vi "Main VERSION 1.1.vi"() -> ()   [LabVIEW 2017]
uses:
  <vilib>/Math Plots/3D Math Plots/3D Surface/3D Surface XCtrl/3D Surface.xctl
  <vilib>/Math Plots/3D Math Plots/3D Surface/3D Surface Datatype/3D Surface Datatype.lvclass
  CSV Reader Inputs.ctl
  Frequency_Type.ctl
  Measurement_Type.ctl
  Digital Channel Selector.ctl
  State.ctl
  Data.ctl
  <vilib>/Platform/TimedLoop/XDataNode/timing_clust.ctl
  <vilib>/Platform/TimedLoop/XDataNode/nitl_modes.ctl
  <vilib>/Platform/TimedLoop/XDataNode/wakeup.ctl
  <vilib>/addons/Control Design/_Model Construction/Data Typedefs.llb/CD DtoC Conversion Method.ctl
  <vilib>/imath/engines/lvmath2/RunTimeEngine/Managers/WorkSpace/UID Generator.vi
  <vilib>/imath/engines/lvmath2/RunTimeEngine/BuiltInFunctions/zpk_to_tf/NIMS_zpk_to_tf.vi
  <vilib>/imath/engines/lvmath2/RunTimeEngine/RunTimeType/NIMS_RunTimeType_From StrictType (excl LVString).vi
  <instcachedir>/0/NIMS_RunTimeType_From StrictType (excl LVString)_DC56D72BB6B948F98D63F1A957D87C42.lvgen/NIMS_RunTimeType_From StrictType (excl LVString)_DC56D72BB6B948F98D63F1A957D87C42_000.vi
  <vilib>/imath/engines/lvmath2/RunTimeEngine/ErrorHandling/NIMS_Error From Error Code.vi
  <vilib>/imath/engines/lvmath2/RunTimeEngine/LocalVariableDefStatement/MC_LocalVariableDefStatement_Display.vi
  <vilib>/imath/engines/lvmath2/RunTimeEngine/Managers/SymbolTable/Clear UID.vi
  <vilib>/imath/engines/lvmath2/RunTimeEngine/NodeEndStatement/NIMS_NodeEndStatement_Output.vi
  <instcachedir>/0/NIMS_NodeEndStatement_Output_53EC0D466D134D7ABD903AC30B43404B.lvgen/NIMS_NodeEndStatement_Output_53EC0D466D134D7ABD903AC30B43404B_005.vi
  <vilib>/imath/engines/lvmath2/RunTimeEngine/ErrorHandling/NIMS_Finalize Error.vi
  <vilib>/addons/Control Design/_Model Construction/Model Creation.llb/Model Creation SubVI/cd_Create Transfer Function Model.vi
  <vilib>/addons/Control Design/_Model Construction/Model Information.llb/Model Information SubVIs/cd_Set Names To TF Model.vi
  <vilib>/addons/Control Design/_Utility/Model Viewer.llb/Model Viewer SubVI/cd_Draw Transfer Function Equation (TF).vi
  <vilib>/addons/Control Design/_Time Response Analysis/Time Response.llb/Time Response subVI/cd_Linear Simulation (Transfer Function).vi
  <vilib>/addons/Control Design/_Dynamic Analysis/Dynamic Analysis.llb/Dynamic Analysis subVI/cd_Damping Ratio and Natural Frequency (Transfer Function).vi
  <vilib>/addons/Wavelet Analysis/application.llb/WA Detrend (Waveform).vi
  Program Files (x86)/National Instruments/LabVIEW 2017/vi.lib/addons/System Identification/Data Preprocess.llb/SI Lowpass Filter (SISO Waveform).vi
  <vilib>/addons/Time Series Analysis/Modeling and Prediction.llb/TSA ARMA Modeling (Waveform).vi
  <vilib>/addons/Control Design/_Model Conversions/Continuous and Discrete.llb/Continuous and Discrete SubVI/cd_Convert Discrete to Continuous (TF).vi
  <vilib>/addons/Control Design/_Model Conversions/Model Type.llb/Model Conversion SubVI/cd_Convert Transfer Function to State-Space Model.vi
  <vilib>/addons/Control Design/_Dynamic Analysis/Dynamic Analysis.llb/Dynamic Analysis subVI/cd_Damping Ratio and Natural Frequency (State-Space).vi
  <vilib>/imath/engines/lvmath2/RunTimeEngine/BuiltInFunctions/sort/NIMS_[2o]_sort(RRowV,I32,Str).vi
  <instcachedir>/0/NIMS_[2o]_sort(RRowV,I32,Str)_E84E23B068DF4763991B1E74560868DE.lvgen/NIMS_[2o]_sort(RRowV,I32,Str)_E84E23B068DF4763991B1E74560868DE_000.vi
  <vilib>/imathl/engines/lvmath/Functions/Error Handling/Create Error.vi
  <vilib>/imath/engines/lvmath2/RunTimeEngine/IndexRead/NIMS V(V).vi
  <instcachedir>/0/NIMS V(V)_298D9CB7BFEB42B8BC8D9C3C28AE8C70.lvgen/NIMS V(V)_298D9CB7BFEB42B8BC8D9C3C28AE8C70_000.vi
  <instcachedir>/0/NIMS V(V)_298D9CB7BFEB42B8BC8D9C3C28AE8C70.lvgen/NIMS V(V)_298D9CB7BFEB42B8BC8D9C3C28AE8C70_001.vi
  <vilib>/imath/engines/lvmath2/RunTimeEngine/BitwiseOperatorToken/NIMS_Bitwise_Operator_And.vi
  <instcachedir>/0/NIMS_Bitwise_Operator_And_BF79565AECDF4B89921EA9614C6BB008.lvgen/NIMS_Bitwise_Operator_And_BF79565AECDF4B89921EA9614C6BB008_001.vi
  <vilib>/imath/engines/lvmath2/RunTimeEngine/BuiltInFunctions/imag/NIMS_imag(Complex).vi
  <instcachedir>/0/NIMS_imag(Complex)_3180D40D00C843A49C2B33397F857BF3.lvgen/NIMS_imag(Complex)_3180D40D00C843A49C2B33397F857BF3_002.vi
  <vilib>/imath/engines/lvmath2/RunTimeEngine/BuiltInFunctions/findnz/NIMS_[1o]_findnz(GRowV).vi
  <instcachedir>/0/NIMS_[1o]_findnz(GRowV)_4566141FE5BA40B7B10E18ED0AB78B2D.lvgen/NIMS_[1o]_findnz(GRowV)_4566141FE5BA40B7B10E18ED0AB78B2D_000.vi
  <vilib>/imath/engines/lvmath2/RunTimeEngine/ErrorHandling/NIMS_Create Error From Enums.vi
  <instcachedir>/0/NIMS_NodeEndStatement_Output_53EC0D466D134D7ABD903AC30B43404B.lvgen/NIMS_NodeEndStatement_Output_53EC0D466D134D7ABD903AC30B43404B_000.vi
  <vilib>/addons/Time Series Analysis/Correlation and Spectral Analysis.llb/TSA ARMA Spectrum (Waveform).vi
  <vilib>/imath/engines/lvmath2/RunTimeEngine/RangeToken/NIMS_Range.vi
  <instcachedir>/0/NIMS_Range_8C005833F4504FD4A29AA23D6150121A.lvgen/NIMS_Range_8C005833F4504FD4A29AA23D6150121A_000.vi
  <vilib>/imath/engines/lvmath2/RunTimeSupport/NIMS_Error if Not Equal.vi
  <instcachedir>/0/NIMS_Error if Not Equal_E5646C1EFB50404BB0542B8CFB81CE27.lvgen/NIMS_Error if Not Equal_E5646C1EFB50404BB0542B8CFB81CE27_001.vi
  <instcachedir>/0/NIMS_Error if Not Equal_E5646C1EFB50404BB0542B8CFB81CE27.lvgen/NIMS_Error if Not Equal_E5646C1EFB50404BB0542B8CFB81CE27_000.vi
  <vilib>/imath/engines/lvmath2/RunTimeEngine/IndexRead/NIMS V($).vi
  <instcachedir>/0/NIMS V($)_C593F32C7F6B43C7B1793952E292524F.lvgen/NIMS V($)_C593F32C7F6B43C7B1793952E292524F_001.vi
  <vilib>/imath/engines/lvmath2/RunTimeEngine/IndexReplace/NIMS M(S,$)=V.vi
  <instcachedir>/0/NIMS M(S,$)=V_552265ADF67C4F4FB07E91CD22492551.lvgen/NIMS M(S,$)=V_552265ADF67C4F4FB07E91CD22492551_000.vi
  <vilib>/imath/engines/lvmath2/RunTimeEngine/IndexReplace/NIMS V(S)=S.vi
  <instcachedir>/0/NIMS V(S)=S_EDDEB2B900FD4B108B325BCE58B17C3D.lvgen/NIMS V(S)=S_EDDEB2B900FD4B108B325BCE58B17C3D_000.vi
  <vilib>/imath/engines/lvmath2/RunTimeEngine/IndexReplace/NIMS V(V)=V.vi
  <instcachedir>/0/NIMS V(V)=V_ACB9F458E2974419B362D656D10048D7.lvgen/NIMS V(V)=V_ACB9F458E2974419B362D656D10048D7_000.vi
  <vilib>/imath/engines/lvmath2/RunTimeEngine/IndexRead/NIMS M(V,$).vi
  <instcachedir>/0/NIMS M(V,$)_21A5155762F74C04AE4EA67BEE0D3EF5.lvgen/NIMS M(V,$)_21A5155762F74C04AE4EA67BEE0D3EF5_004.vi
  <instcachedir>/0/NIMS_NodeEndStatement_Output_53EC0D466D134D7ABD903AC30B43404B.lvgen/NIMS_NodeEndStatement_Output_53EC0D466D134D7ABD903AC30B43404B_009.vi
  <instcachedir>/0/NIMS_NodeEndStatement_Output_53EC0D466D134D7ABD903AC30B43404B.lvgen/NIMS_NodeEndStatement_Output_53EC0D466D134D7ABD903AC30B43404B_002.vi
  <instcachedir>/0/NIMS_NodeEndStatement_Output_53EC0D466D134D7ABD903AC30B43404B.lvgen/NIMS_NodeEndStatement_Output_53EC0D466D134D7ABD903AC30B43404B_001.vi
  <vilib>/Math Plots/3D Math Plots/3D Surface/3D Surface Datatype/Public/Plot Helper (Vector).vi
  <vilib>/platform/TimedLoop/XDataNode/XDataNode.xnode
  Program Files (x86)/National Instruments/LabVIEW 2017/vi.lib/addons/System Identification/NI_SysID.lvlib
  <vilib>/addons/_Advanced Signal Processing/NI_AdvSigProcWA.lvlib
  <vilib>/addons/_Advanced Signal Processing/NI_AdvSigProcTSA.lvlib
  <vilib>/addons/Control Design/_Model Construction/NI_LinSys_Model Creation.lvlib
  <vilib>/addons/Control Design/_Model Conversions/NI_CD_Continuous and Discrete.lvlib
  <vilib>/addons/Control Design/_Model Construction/NI_LinSys_Data Typedefs.lvlib
  <vilib>/Analysis/NI_AALBase.lvlib
  <vilib>/addons/Control Design/_Dynamic Analysis/NI_CD_Dynamic Analysis.lvlib
  <vilib>/Platform/TimedLoop/XDataNode/XDNodeRunTimeDep.lvlib
  <vilib>/addons/Control Design/_Model Conversions/NI_CD_Model Type.lvlib
  <vilib>/Analysis/NI_AALPro.lvlib
  <vilib>/addons/Control Design/_Time Response Analysis/NI_CD_Time Response.lvlib
  <vilib>/imath/engines/lvmath2/RunTimeEngine/Managers/SymbolTable/NIMS_WorkSpace.lvlib
  <vilib>/addons/Control Design/_Model Construction/NI_LinSys_Model Information.lvlib
  <vilib>/addons/Control Design/_Utility/NI_CD_Model Viewer.lvlib
  <vilib>/S3DK/PMU Recorder Light/PMU Recorder Light.lvlib
panel:
  in  "Tab Control 3":enum32{"Test", "Simulation"}(tab)
  in  "Terminal ID 2 (Phase Comparison)":dbl
  in  "Test Method":enum16{"Use PRL Data", "Read from CSV File"}(ring)
  in  "CSV Reader Inputs":T1={"Frequency Type"=enum."Frequency", "Measurement Type"=enum."Power", "Digital Channel Selector"=enum."2", "Format Type"=enum."Format B", "CSV File Input"=path ""}
  in  "Terminal ID":dbl
  in  "Input Poles":cdb[](array[numeric])
  in  "Input Zeros":cdb[](array[numeric])
  out "Input Transfer Function":picture
  in  "Input Frequency (Hz)":dbl
  in  "Input Damping Ratio (%)":dbl
  in  "Simulation Method":T5(ring)
  out "Poles":cdb[](array[numeric]) format="%.2f"
  out "Damping Ratios (%)":dbl[](array[numeric]) format="%.2f"
  out "Natural Frequencies":dbl[](array[numeric]) format="%.2f"
  in  "Tab Control":enum32{"Data", "Preprocessed Data"}(tab)
  out "Real-time data":waveform(dbl)(graph)={"t0"=timestamp(3467964116.0127993 s since 1904-01-01), "dt"=0.02, "Y"=array[30000 elements]}
  out "Preprocessed data":waveform(dbl)(graph)={"t0"=timestamp(3467964116.0127993 s since 1904-01-01), "dt"=0.2, "Y"=array[3000 elements]}
  in  "Tab Control 2":T6(tab)=enum."Options"
  out "Critical Damping [%]":dbl
  out "Critical Frequency [Hz]":dbl
  out "Estimated Complex Plane":cluster{dbl[], dbl[]}(graph)
  out "Damping ratio evolution":dbl[][](graph)
  in  "Number of critical modes":i32=1
  in  "Length of Spectra [s]":dbl=12.0
  out "Spectrogram":refnum<class "3D Plot Datatype.lvclass">[](xcontrol)
  in  "dB Scale":bool=TRUE
  out "Spectrum":cluster{"f0":dbl, "df":dbl, "S(f)":dbl[]}(graph)={"f0"=0.0, "df"=0.0048828125, "S(f)"=[]}
  out "ARMA Transfer Function":picture
  out "Picture 9":picture
  out "Picture 8":picture
  out "Picture 7":picture
  out "Picture 6":picture
  out "Picture 5":picture
  out "Picture 4":picture
  out "Picture 3":picture
  out "Picture 2":picture
  out "Picture 1":picture
  out "Std of Damping":dbl[](array[numeric])=[3.167813045881809]
  out "Mean Damping [%]":dbl[](array[numeric])=[5.49924934647624]
  out "Frequency[Hz]":dbl[](array[numeric])=[1.626086044993813, 0.5198061588603065, 1.9739015777045272] format="%.4f"
  out "Damping Ratio [%]":dbl[](array[numeric])=[11.530156484123282, 15.381771713903165, 15.639879258359347] format="%.4f"
  out "Complex Poles":cdb[](array[numeric])=[-1.1780360817698377+10.148858009104277i, -0.5023745738423925+3.227170083530164i, -1.9397187258807729+12.249765461704891i] format="%.4f"
  in  "Upper Damping [%]":dbl=20.0
  in  "Lower Damping [%]":dbl
  in  "Upper Frequency [Hz]":dbl=2.0
  in  "Lower Frequency [Hz]":dbl=0.08
  in  "Signal Selection":T7(radio)=enum."Analog"
  in  "Downsampling Ratio":dbl=1.0
  in  "LPF Cut-off Frequency [Hz]":dbl=2.5
  in  "Low-Pass Filter Order":i32=5
  in  "Detrend Cut-off Frequency (Hz)":dbl=0.05
  in  "MA Order":i32=10
  in  "Sampling Frequency (Hz)":dbl=50.0
  in  "AR Order":i32=25
  in  "Parcel Length (Simulation)":i32=30000
  in  "Refresh Rate [s]":i32=10
  in  "Std Threshold":dbl=1.35
  out "Parcel Length (SDK or Simulation)":i32=30000
  in  "Simulate Data?":bool
  out "Simulation":bool
  in  "stop":bool
  # "Simulated Expected Values"
  # "NOTE: If using PRL Data, you must have the S3DK GUI and\nchannel selector enabled from another VI (i.e. Test PDC)"
  # "**Must enter CSV file before running"
  # "***Has the ability to shows more than 1 graph based on parameters\n\n- Each row of data (numerical results) equates to 1 mode"
  # "MA\n_______\n\n   AR"
  # "Note: Phase Comparison cannot be used for Format A\n since the data is only for 1 terminal"
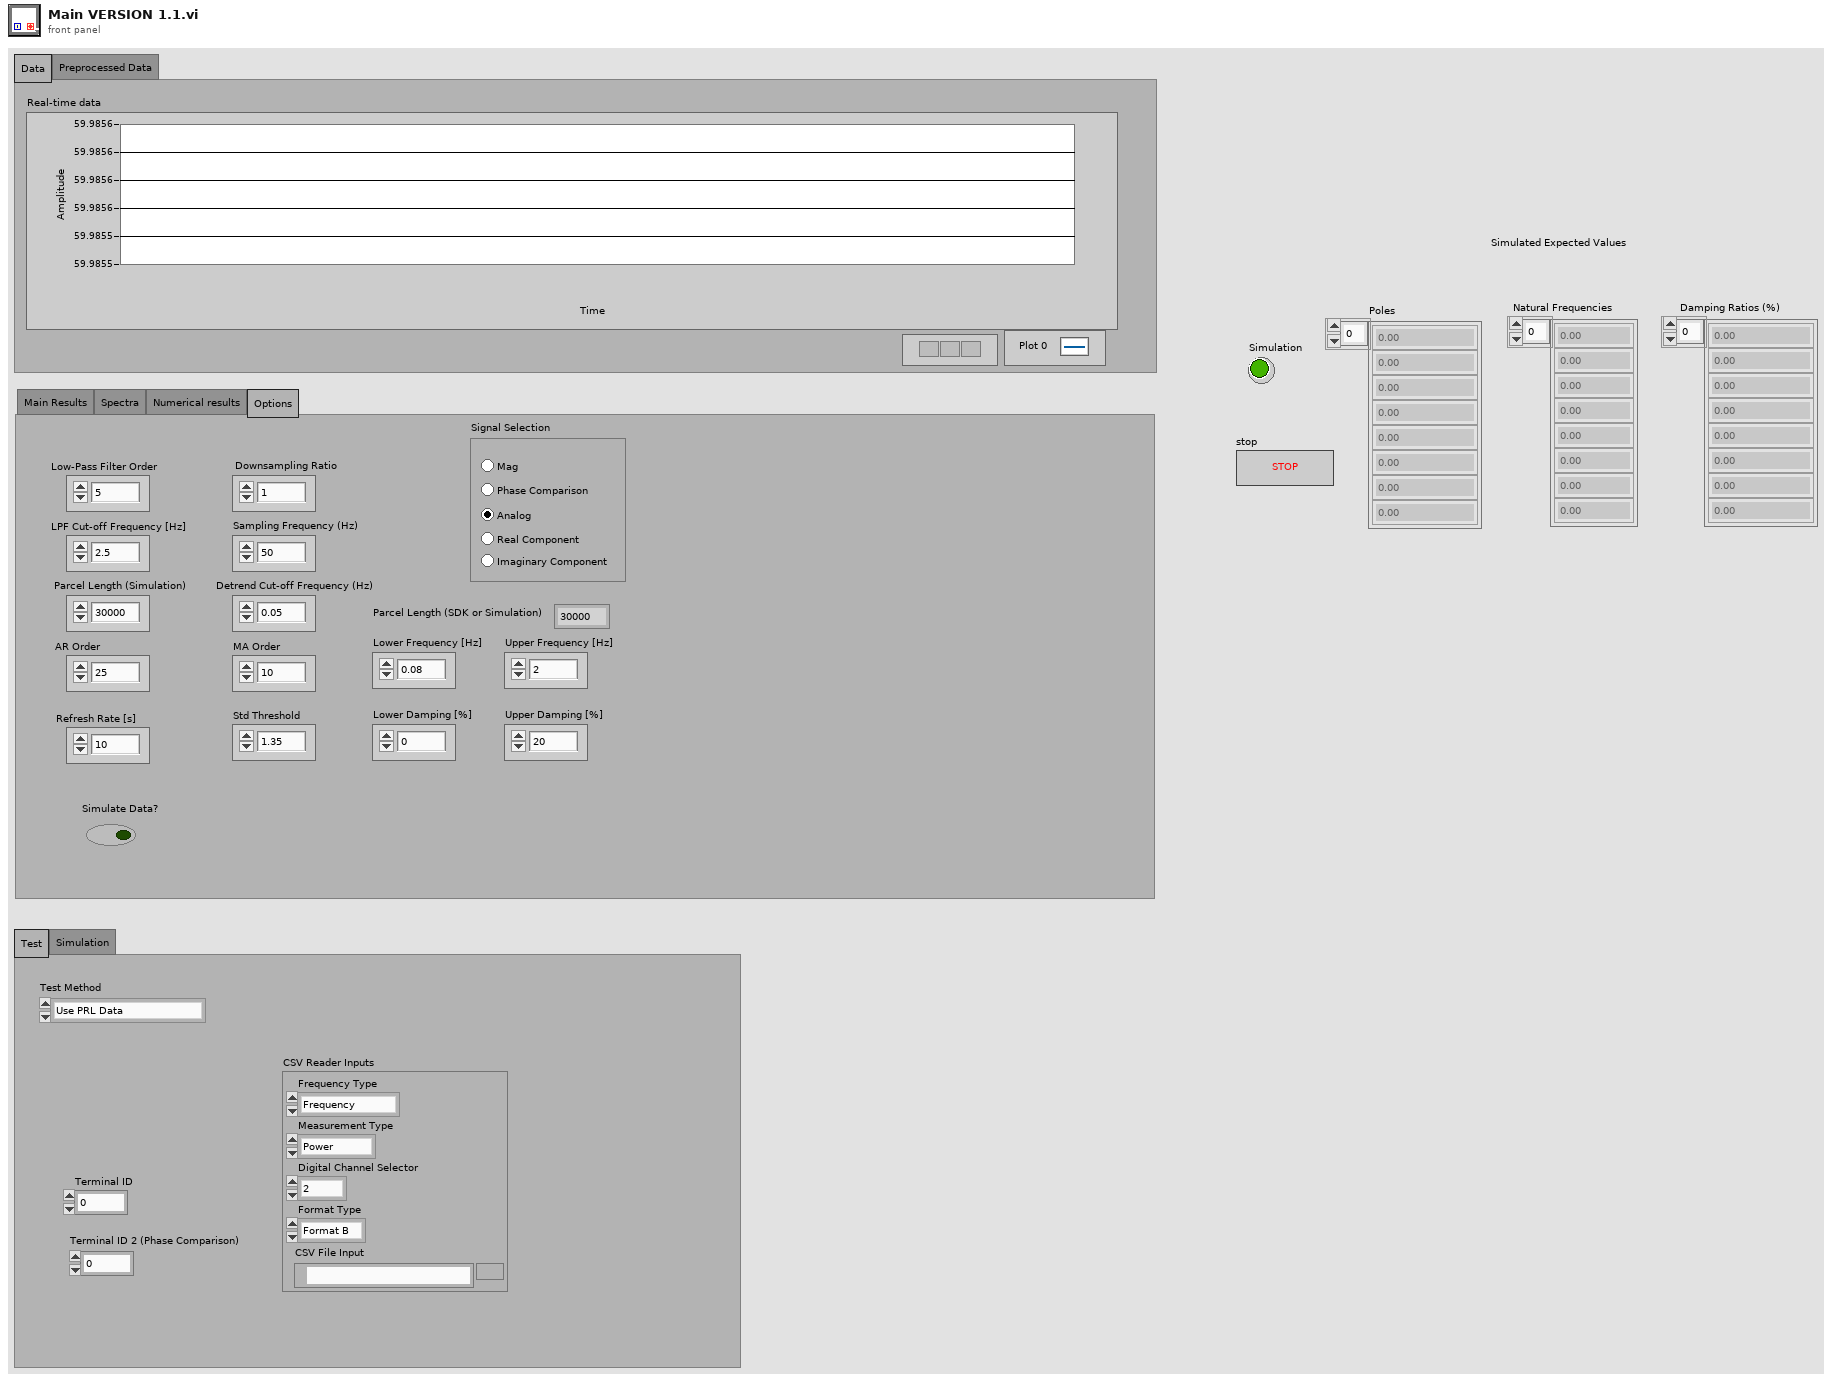
[diagram p1: front panel]
types:
  T1 = typedef "CSV Reader Inputs.ctl" = cluster{"Frequency Type":T2, "Measurement Type":T3, "Digital Channel Selector":T4, "Format Type":enum16{"Format A", "Format B"}, "CSV File Input":path}
  T2 = typedef "Frequency_Type.ctl" = enum16{"Frequency", "df/dt"}
  T3 = typedef "Measurement_Type.ctl" = enum16{"Voltage", "Current", "Power"}
  T4 = typedef "Digital Channel Selector.ctl" = enum16{"1", "2", "3"}
  T5 = enum16{"Use Input Frequency/D.R.", "Use Input Poles/Zeroes"}
  T6 = enum32{"Main Results", "Spectra", "Numerical results", "Options"}
  T7 = enum32{"Mag", "Phase Comparison", "Analog", "Real Component", "Imaginary Component"}
  T8 = enum8{"Enabled", "Disabled", "Disabled and Grayed Out"}
  T9 = typedef "data.ctl" = cluster{"Waveform":waveform(dbl), "Parcel Length":i32, "AR Order":i32, "Sampling Frequency":dbl, "MA Order ":i32}
  T10 = typedef "State.ctl" = enum16{"Initialize", "Read Real Data", "Read Simulated Data", "Preprocessing", "Compute AR/MA Coeffs", "Get Spectrum"}
  T11 = typedef "XDNodeRunTimeDep.lvlib/timing_clust.ctl" = cluster{"Expected End [f-1]":u64, "Actual End [f-1]":u64, "Finished Late? [f-1]":bool, "Expected End [i-1]":u64, "Actual End [i-1]":u64, "Finished Late? [i-1]":bool, "Expected Start [i]":u64, "Actual Start [i]":u64, "Expected Start [f]":u64, "Actual Start [f]":u64, "Source Name":string, "Structure Name":string, "Period":i64, "Deadline":i64, "Offset":i64, "Start":i64, "Priority":i32, "Timeout":i32, "Mode":T12, "Wakeup Reason":T13, "Error":errorcluster, "Source Type":string, "Secondary Source Type":string, "Global End Time":u64, "Global Start Time":u64, "Frame Duration":u64, "Iteration Duration":u64, "Assigned CPU":i32, "I/O Scan Engine Mode":u32}
  T12 = typedef "XDNodeRunTimeDep.lvlib/nitl_modes.ctl" = enum32{"No Change", "Process missed periods, maintain original phase", "Discard missed periods, maintain original phase", "Process missed periods, ignore original phase", "Discard missed periods, ignore original phase"}
  T13 = typedef "XDNodeRunTimeDep.lvlib/wakeup.ctl" = enum32{"Normal", "Aborted", "Asynchronous wakeup", "Timing source error", "Timed loop error", "Timeout"}
  T14 = cluster{"Timestamps":timestamp[], "Phasor Data":cdb[], "Analog Data":dbl[], "Phasor Data 2":cdb[]}
  T15 = typedef "Terminal Data v1.ctl" = cluster{"Terminal Name":string, "Terminal ID":dbl, "Timestamps":timestamp[], "Phasor Data":cdb[], "Analog Data":dbl[], "Status":dbl[], "Digital Data":dbl[]}
  T16 = typedef "NI_LinSys_Model Typedefs.lvlib/CD Transfer Function Model (MIMO).ctl" = cluster{"properties":T17, "transfer function(s)":T18[][]}
  T17 = typedef "NI_LinSys_Model Typedefs.lvlib/CD General Elements.ctl" = cluster{"Model name":string, "Input names":string[], "Output names":string[], "Input Delays":dbl[], "Output Delays":dbl[], "Sampling Time":dbl, "Notes":string}
  T18 = typedef "NI_LinSys_Model Typedefs.lvlib/CD Transfer Function Model (SISO).ctl" = cluster{"Numerator":dbl[], "Denominator":dbl[], "delay":dbl}
  T19 = typedef "NI_LinSys_Data Typedefs.lvlib/CD MIMO Time Response Data.ctl" = cluster{"Time":dbl[], "Outputs Data":dbl[][][], "States Data":dbl[][][], "plot type":T20}
  T20 = typedef "NI_LinSys_Data Typedefs.lvlib/CD Plot Types Enum.ctl" = enum16{"bode-magnitude", "bode-phase", "nichols", "nyquist", "singular values", "step", "impulse", "initial", "simulation", "nyquist with separation"}
  T21 = typedef "NI_LinSys_Data Typedefs.lvlib/CD DtoC Conversion Method.ctl" = u16
  T22 = typedef "NI_LinSys_Model Typedefs.lvlib/CD State Space Model (MIMO).ctl" = cluster{"properties":T17, "A":dbl[][], "B":dbl[][], "C":dbl[][], "D":dbl[][], "StateNames":string[], "Transport Delay":dbl[][]}
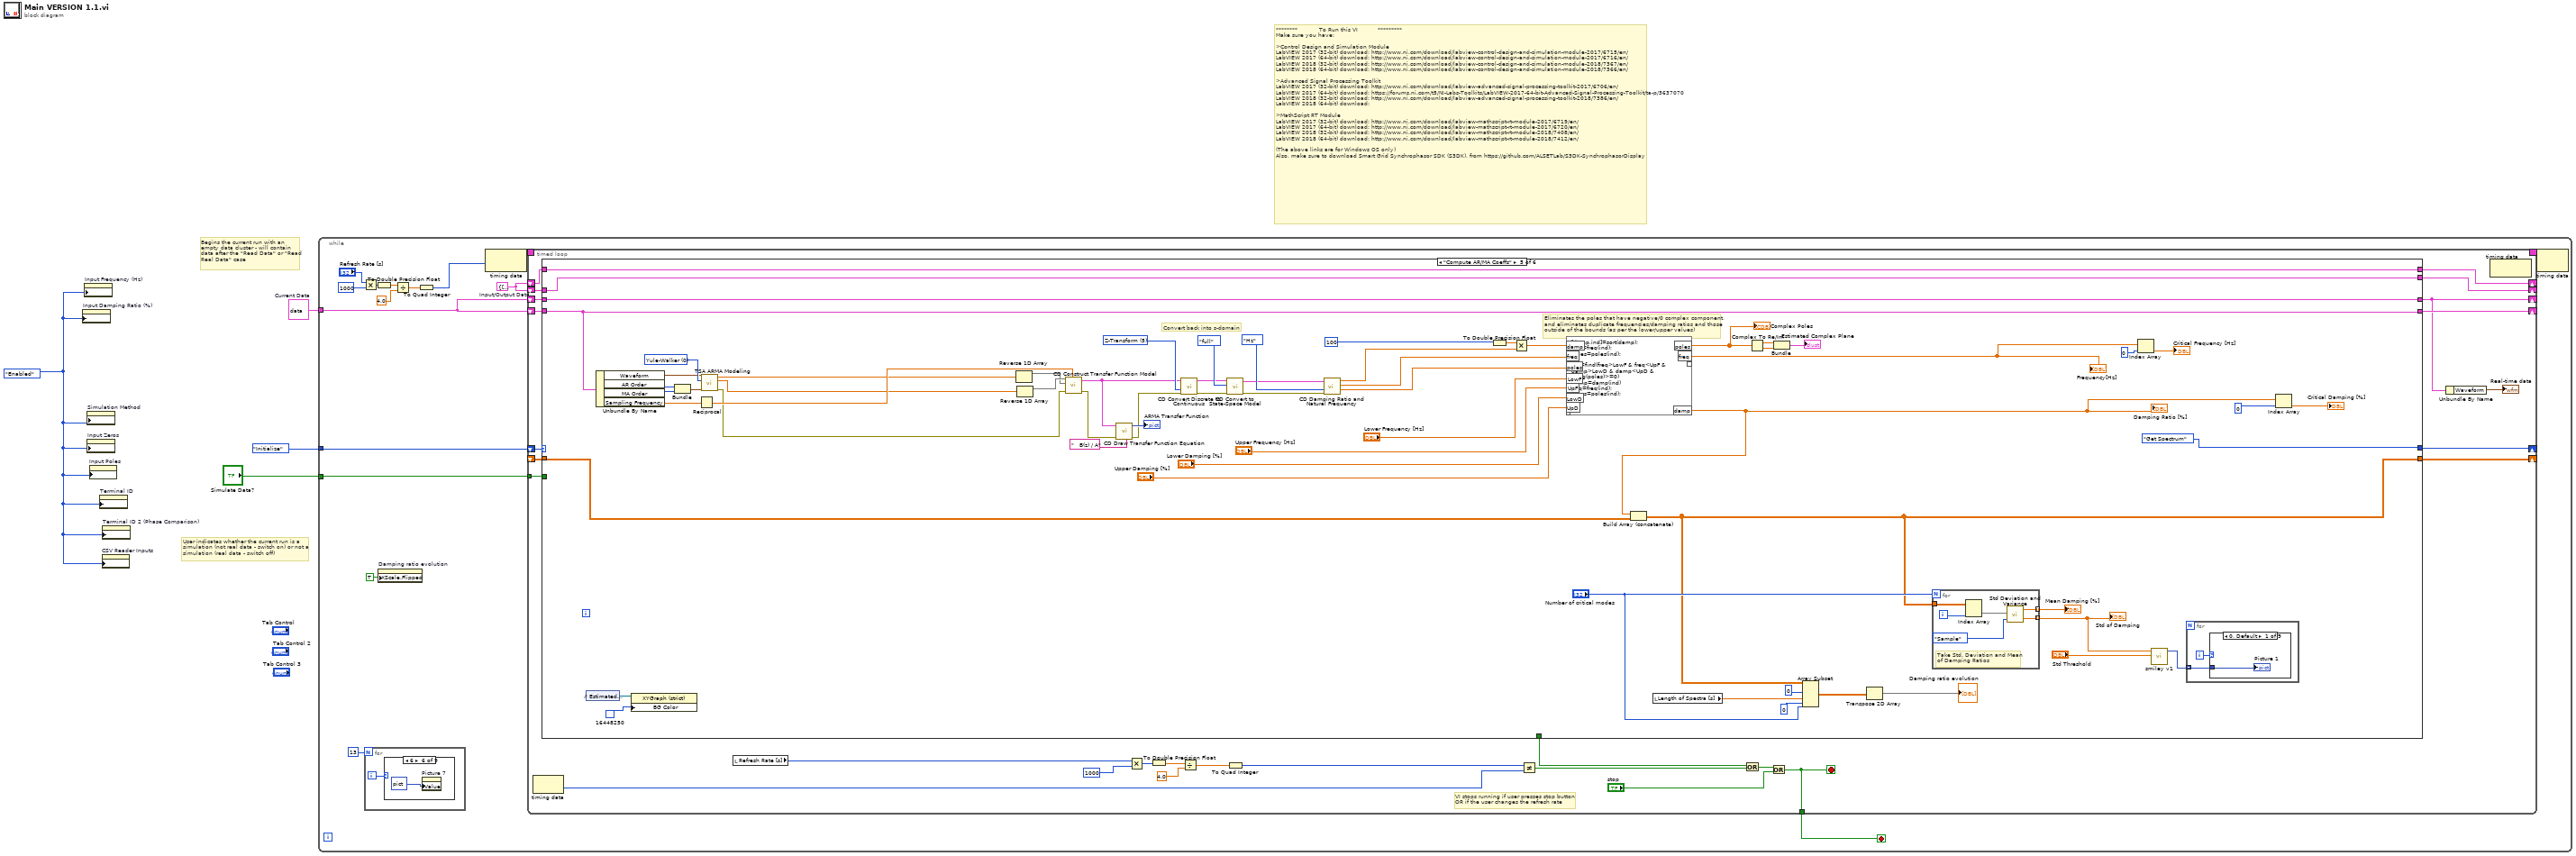
[diagram p0: block diagram]
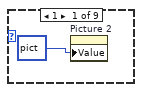
[diagram p2: hidden frame]
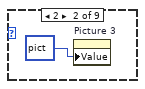
[diagram p3: hidden frame]
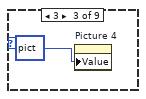
[diagram p4: hidden frame]
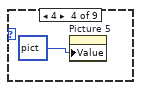
[diagram p5: hidden frame]
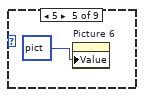
[diagram p6: hidden frame]
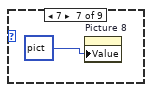
[diagram p7: hidden frame]
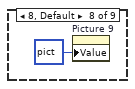
[diagram p8: hidden frame]
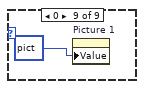
[diagram p9: hidden frame]
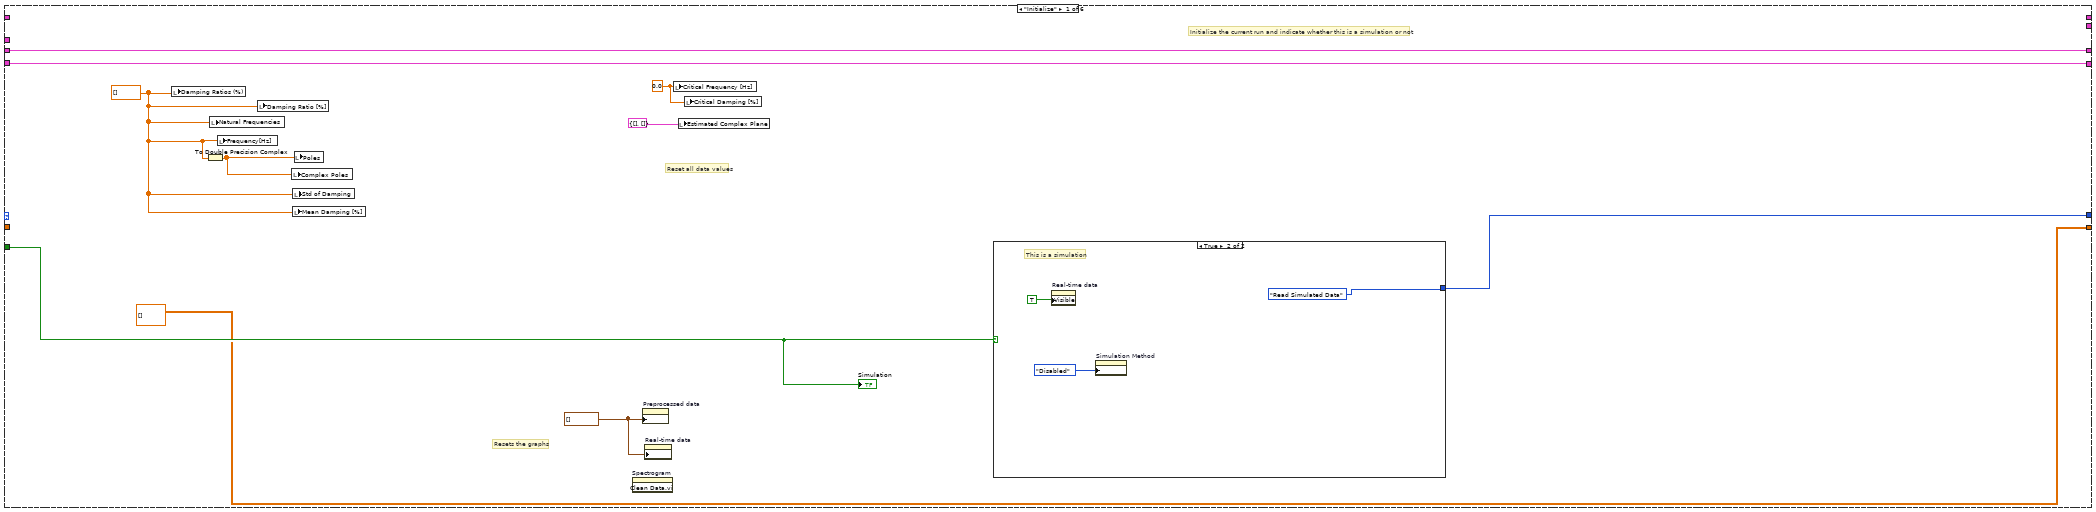
[diagram p10: hidden frame]
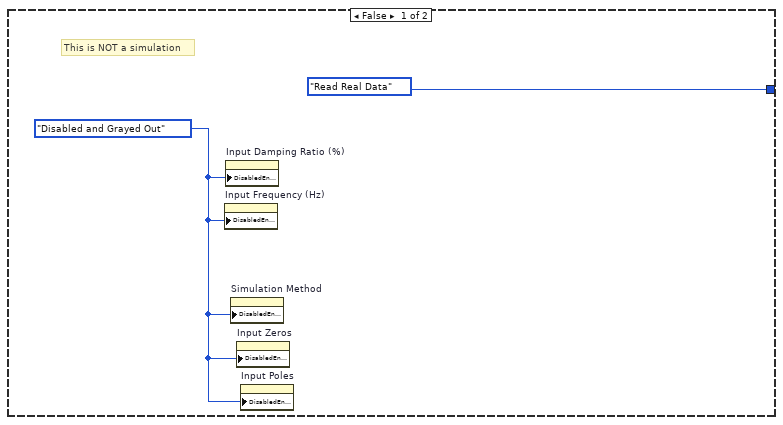
[diagram p11: hidden frame]
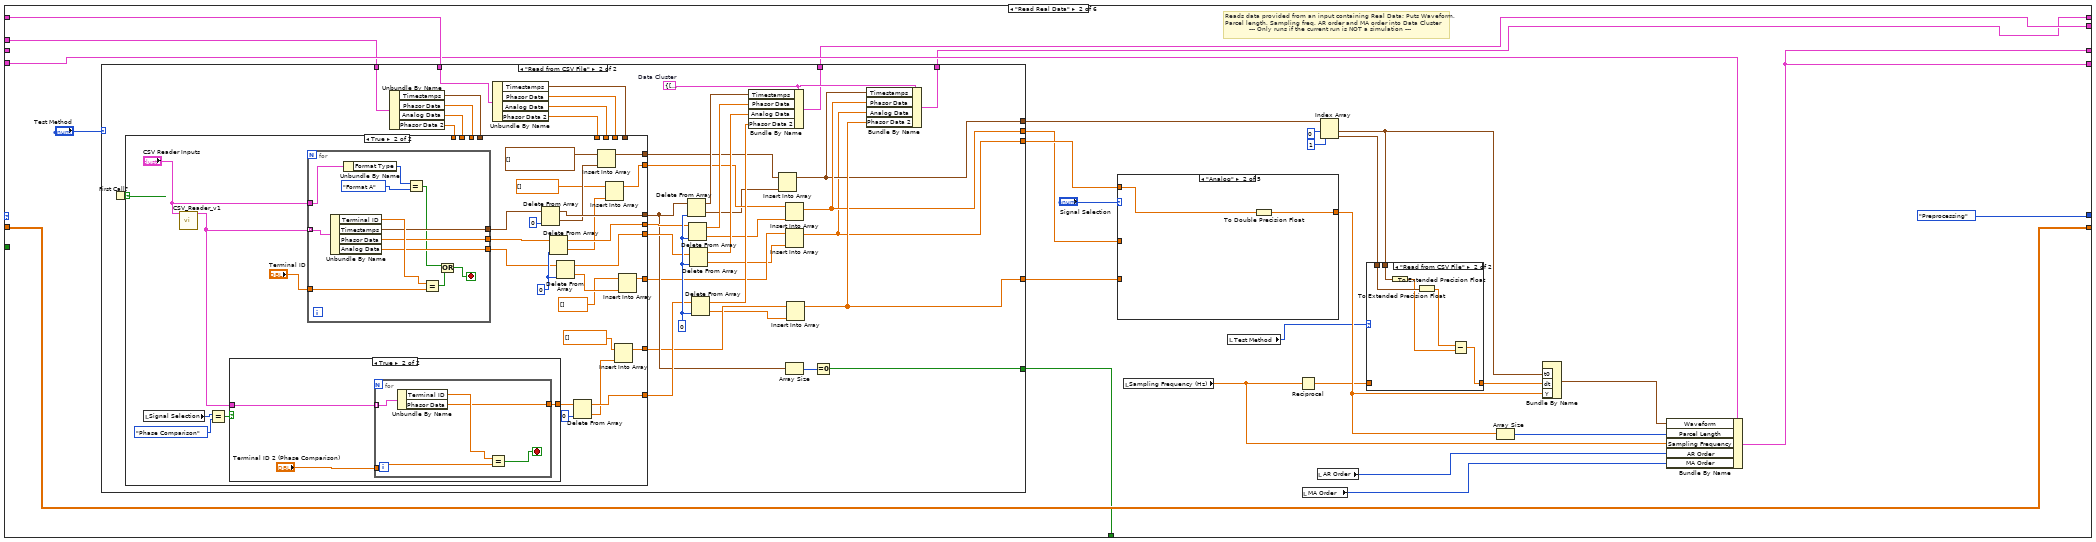
[diagram p12: hidden frame]
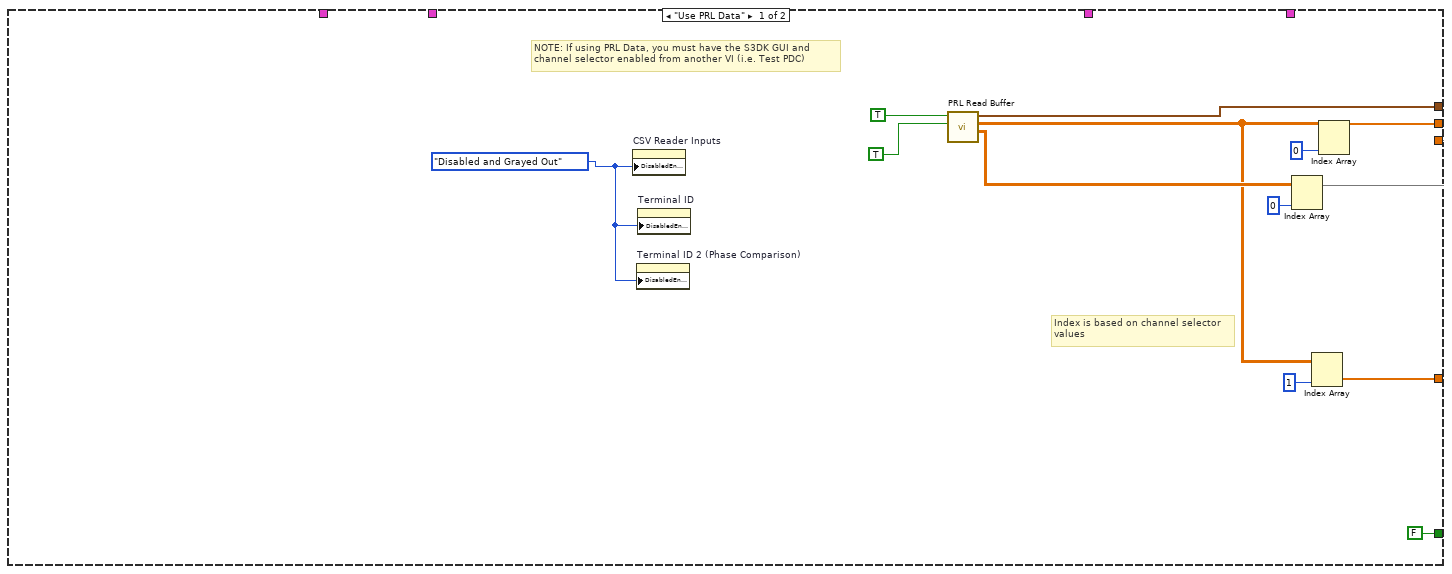
[diagram p14: hidden frame]
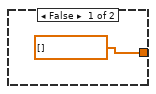
[diagram p16: hidden frame]
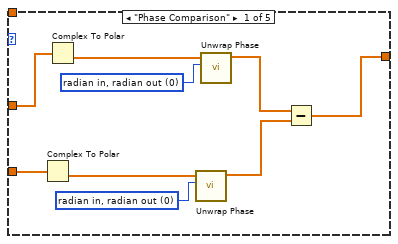
[diagram p17: hidden frame]
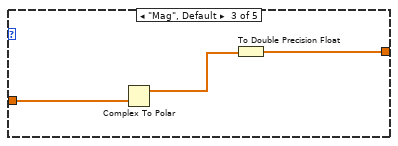
[diagram p18: hidden frame]
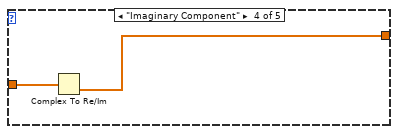
[diagram p19: hidden frame]
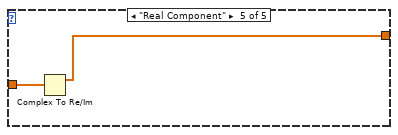
[diagram p20: hidden frame]
diagram:
  w1 = T8."Enabled" ("Disabled")
  w3 = T9 {"Waveform"={"t0"=timestamp(0 s since 1904-01-01), "dt"=1.0, "Y"=[]}, "Parcel Length"=0, "AR Order"=0, "Sampling Frequency"=0.0, "MA Order "=0}  # Current Data
  # "Begins the current run with an \nempty data cluster - will contain\ndata after the \"Read Data\" or \"Read \nReal Data\" case"
  # "User indicates whether the current run is a \nsimulation (not real data - switch on) or not a\nsimulation (real data - switch off)"
  # "********            To Run this VI           *********\nMake sure you have:\n\n>Control Design and Simulation Module\nLabVIEW 2017 (32-bit) download: http://www.ni.com/download/labview-control-design-and-simulation-module-2017/6715/en/\nLabVIEW 2017 (64-bit) download: http://www.ni.com/download/labview-control-design-and-simulation-module-2017/6716/en/ \nLabVIEW 2018 (32-bit) download: http://www.ni.com/download/labview-control-design-and-simulation-module-2018/7367/en/\nLabVIEW 2018 (64-bit) download: http://www.ni.com/download/labview-control-design-and-simulation-module-2018/7366/en/\n\n>Advanced Signal Processing Toolkit\nLabVIEW 2017 (32-bit) download: http://www.ni.com/download/labview-advanced-signal-processing-toolkit-2017/6706/en/\nLabVIEW 2017 (64-bit) download: https://forums.ni.com/t5/NI-Labs-Toolkits/LabVIEW-2017-64-bit-Advanced-Signal-Processing-Toolkit/ta-p/3637070\nLabVIEW 2018 (32-bit) download: http://www.ni.com/download/labview-advanced-signal-processing-toolkit-2018/7386/en/\nLabVIEW 2018 (64-bit) download:\n\n>MathScript RT Module\nLabVIEW 2017 (32-bit) download: http://www.ni.com/download/labview-mathscript-rt-module-2017/6719/en/\nLabVIEW 2017 (64-bit) download: http://www.ni.com/download/labview-mathscript-rt-module-2017/6720/en/ \nLabVIEW 2018 (32-bit) download: http://www.ni.com/download/labview-mathscript-rt-module-2018/7408/en/\nLabVIEW 2018 (64-bit) download: http://www.ni.com/download/labview-mathscript-rt-module-2018/7412/en/ \n\n(The above links are for Windows OS only)\nAlso, make sure to download Smart Grid Synchrophasor SDK (S3DK), from https://github.com/ALSETLab/S3DK-SynchrophasorDisplay"
  n1 = property on="Input Damping Ratio (%)" class="DigNum (strict)"("DisabledEnum"=w1) -> ()  [unwired: 2 in, 2 out]
  n2 = property on="Input Frequency (Hz)" class="DigNum (strict)"("DisabledEnum"=w1) -> ()  [unwired: 2 in, 2 out]
  n3 = property on="Simulation Method" class="Enum (strict)"("DisabledEnum"=w1) -> ()  [unwired: 2 in, 2 out]
  n4 = property on="Input Zeros" class="Arr (strict)"("DisabledEnum"=w1) -> ()  [unwired: 2 in, 2 out]
  n5 = property on="Input Poles" class="Arr (strict)"("DisabledEnum"=w1) -> ()  [unwired: 2 in, 2 out]
  n6 = property on="Terminal ID" class="DigNum (strict)"("DisabledEnum"=w1) -> ()  [unwired: 2 in, 2 out]
  n7 = property on="CSV Reader Inputs" class="Clust (strict)"("DisabledEnum"=w1) -> ()  [unwired: 2 in, 2 out]
  n8 = property on="Terminal ID 2 (Phase Comparison)" class="DigNum (strict)"("DisabledEnum"=w1) -> ()  [unwired: 2 in, 2 out]
  n9 = while {
    tunnel: State."Initialize" ("Enum") -> [w7]
    tunnel: w3 -> [w8]
    tunnel: "Simulate Data?" -> [w12]
    stop <- w5 stop-if-true
    w6 = T14 {"Timestamps"=[], "Phasor Data"=[], "Analog Data"=[], "Phasor Data 2"=[]}  # Input/Output Data
    n10 = Multiply(x="Refresh Rate [s]", y=1000) -> (x*y=w9:i32)
    n11 = for {
      N: 13 -> [_]
      i -> [w21]
      n12 = case shown="6" w21 {
        frame 1 {
          n13 = property on="Picture 2" class="Pict"("Value"=picture bytes[260130] ("Picture 9")) -> ()  [unwired: 2 in, 2 out]
        }
        frame 2 {
          n14 = property on="Picture 3" class="Pict"("Value"=picture bytes[260130] ("Picture 9")) -> ()  [unwired: 2 in, 2 out]
        }
        frame 3 {
          n15 = property on="Picture 4" class="Pict"("Value"=picture bytes[260130] ("Picture 9")) -> ()  [unwired: 2 in, 2 out]
        }
        frame 4 {
          n16 = property on="Picture 5" class="Pict"("Value"=picture bytes[260130] ("Picture 9")) -> ()  [unwired: 2 in, 2 out]
        }
        frame 5 {
          n17 = property on="Picture 6" class="Pict"("Value"=picture bytes[260130] ("Picture 9")) -> ()  [unwired: 2 in, 2 out]
        }
        frame 6 {
          n18 = property on="Picture 7" class="Pict"("Value"=picture bytes[260130] ("Picture 9")) -> ()  [unwired: 2 in, 2 out]
        }
        frame 7 {
          n19 = property on="Picture 8" class="Pict"("Value"=picture bytes[260130] ("Picture 9")) -> ()  [unwired: 2 in, 2 out]
        }
        frame 8, Default {
          n20 = property on="Picture 9" class="Pict"("Value"=picture bytes[260130] ("Picture 9")) -> ()  [unwired: 2 in, 2 out]
        }
        frame 0 {
          n21 = property on="Picture 1" class="Pict"("Value"=picture bytes[260130] ("Picture 9")) -> ()  [unwired: 2 in, 2 out]
        }
      }
    }
    n22 = To Double Precision Float(number=w9) -> (double precision float=w10:dbl)
    n23 = property on="Damping ratio evolution" class="WFGraph (strict)"("XScale.Flipped"=TRUE ("X Scale.Flipped")) -> ()  [unwired: 2 in, 2 out]
    n24 = Divide(x=w10, y=4.0) -> (x/y=w15:dbl)
    n25 = To Quad Integer(1:w15) -> (0:w14:i64)
    n26 = node-c288(w14) -> (w20:T11)
    n27 = timed-loop {
      shift-right: [w46] -> _
      shift-left: w8 -> [w57]
      shift-right: [w39] -> _
      shift-left: w7 -> [w40]
      timing: w20 -> [_]
      timing-out: [_] -> w19
      shift-right: [w49] -> _
      shift-left: _ -> [w48]
      tunnel: w12 -> [w47]
      shift-right: [w44] -> _
      shift-left: w8 -> [w43]
      shift-right: [w37] -> _
      shift-left: w6 -> [w38]
      shift-right: [w36] -> _
      shift-left: w6 -> [w35]
      tunnel: [w34] -> w5
      stop <- w34 stop-if-true
      # "VI stops running if user presses stop button\nOR if the user changes the refresh rate"
      n28 = node-c288() -> (w56:i64)  [unwired: 1 in]
      n29 = case shown="\"Compute AR/MA Coeffs\"" w40 {
        tunnel: w57 -> [w70 w86 w273 w371 w442 w700]
        tunnel: [w70 w96 w265 w380 w442 w700] -> w46
        tunnel: [dbl[][] [] w98 w266 w372 w402 w696] -> w49
        tunnel: w48 -> [_ w98 w266 w372 w432 w696]
        tunnel: w47 -> [w64 _ _ _ _ _]
        tunnel: [w69 w96 w265 w370 w424 w692] -> w44
        tunnel: w43 -> [w69 _ _ w370 w424 w692]
        tunnel: [w62 State."Preprocessing" ("Enum") State."Preprocessing" ("Enum") State."Compute AR/MA Coeffs" ("Enum") State."Get Spectrum" ("Enum") w681] -> w39
        tunnel: [_ w83 _ w366 w385 w678] -> w37
        tunnel: w38 -> [_ w87 _ w366 w385 w678]
        tunnel: [_ w84 _ w362 w381 w677] -> w36
        tunnel: w35 -> [_ w85 _ w362 w381 w677]
        tunnel: [_ w82 _ _ _ _] -> w32
        frame "Initialize" {
          w65 = 0.0 ("Critical Frequency [Hz]")
          w67 = waveform(dbl)[] [] ("History Data")
          w63 = dbl[] [] ("Array - Numeric")
          # "Reset all data values"
          # "Resets the graphs"
          # "Initialize the current run and indicate whether this is a simulation or not"
          n30 = local write "Damping Ratios (%)"(w63) -> ()
          n31 = To Double Precision Complex(1:w63) -> (0:w68:cdb[])
          n32 = local write "Natural Frequencies"(w63) -> ()
          n33 = local write "Frequency[Hz]"(w63) -> ()
          n34 = local write "Damping Ratio [%]"(w63) -> ()
          n35 = local write "Complex Poles"(w68) -> ()
          n36 = local write "Mean Damping [%]"(w63) -> ()
          n37 = local write "Std of Damping"(w63) -> ()
          n38 = local write "Poles"(w68) -> ()
          n39 = invoke on="Spectrogram" class="3D Surface (strict)" method="Clean Data.vi"() -> ()  [unwired: 3 in, 3 out]
          n40 = property on="Preprocessed data" class="WFChart (strict)"("History Data"=w67) -> ()  [unwired: 2 in, 2 out]
          n41 = property on="Real-time data" class="WFChart (strict)"("History Data"=w67) -> ()  [unwired: 2 in, 2 out]
          n42 = local write "Critical Frequency [Hz]"(w65) -> ()
          n43 = local write "Estimated Complex Plane"(cluster{"Array":dbl[], "Array 2":dbl[]} {"Array"=[], "Array 2"=[]} ("Cluster")) -> ()
          n44 = local write "Critical Damping [%]"(w65) -> ()
          n45 = case shown="True" w64 {
            tunnel: [State."Read Real Data" ("Enum") State."Read Simulated Data" ("Enum")] -> w62
            frame False {
              w72 = T8."Disabled and Grayed Out" ("Disabled")
              # "This is NOT a simulation"
              n46 = property on="Input Frequency (Hz)" class="DigNum (strict)"("DisabledEnum"=w72) -> ()  [unwired: 2 in, 2 out]
              n47 = property on="Input Damping Ratio (%)" class="DigNum (strict)"("DisabledEnum"=w72) -> ()  [unwired: 2 in, 2 out]
              n48 = property on="Simulation Method" class="Enum (strict)"("DisabledEnum"=w72) -> ()  [unwired: 2 in, 2 out]
              n49 = property on="Input Zeros" class="Arr (strict)"("DisabledEnum"=w72) -> ()  [unwired: 2 in, 2 out]
              n50 = property on="Input Poles" class="Arr (strict)"("DisabledEnum"=w72) -> ()  [unwired: 2 in, 2 out]
            }
            frame True {
              # "This is a simulation"
              n51 = property on="Real-time data" class="WFChart (strict)"("Visible"=TRUE) -> ()  [unwired: 2 in, 2 out]
              n52 = property on="Simulation Method" class="Enum (strict)"("DisabledEnum"=T8."Disabled" ("Disabled")) -> ()  [unwired: 2 in, 2 out]
            }
          }
          "Simulation" <- w64
        }
        frame "Read Real Data" {
          # "Reads data provided from an input containing Real Data; Puts Waveform, \nParcel length, Sampling freq, AR order and MA order into Data Cluster \n            --- Only runs if the current run is NOT a simulation ---"
          n53 = case shown="\"Read from CSV File\"" "Test Method" {
            tunnel: [w122 w128] -> w94
            tunnel: [w117 w131] -> w91
            tunnel: [w115 w125] -> w93
            tunnel: [w112 w132] -> w89
            tunnel: [_ w139] -> w84
            tunnel: w87 -> [_ w153]
            tunnel: [_ w138] -> w83
            tunnel: w85 -> [_ w154]
            tunnel: [FALSE w136] -> w82
            frame "Use PRL Data" {
              w110 = T8."Disabled and Grayed Out" ("Disabled")
              # "NOTE: If using PRL Data, you must have the S3DK GUI and\nchannel selector enabled from another VI (i.e. Test PDC)"
              # "Index is based on channel selector\nvalues"
              n54 = property on="CSV Reader Inputs" class="Clust (strict)"("DisabledEnum"=w110) -> ()  [unwired: 2 in, 2 out]
              n55 = property on="Terminal ID 2 (Phase Comparison)" class="DigNum (strict)"("DisabledEnum"=w110) -> ()  [unwired: 2 in, 2 out]
              n56 = property on="Terminal ID" class="DigNum (strict)"("DisabledEnum"=w110) -> ()  [unwired: 2 in, 2 out]
              n57 = call <vilib>:"PRL Read Buffer .vi"("Get All Signals"=TRUE, "Get Full Buffer"=TRUE) -> ("Analog Signals"=w116:sgl[][], "Phasor Signals"=w113:csg[][], "Timestamp"=w122:timestamp[])  [unwired: 4 in, 3 out]
              n58 = Index Array "Index Array"(array=w116, index (col)=0 ("disabled index (col)")) -> (element=w115:sgl[])  [unwired: 1 in]
              n59 = Index Array "Index Array"(array=w113, index (col)=1 ("disabled index (col)")) -> (element=w112:csg[])  [unwired: 1 in]
              n60 = Index Array "Index Array"(array=w113, index (col)=0 ("disabled index (col)")) -> (element=w117:csg[])  [unwired: 1 in]
            }
            frame "Read from CSV File" {
              w144 = T14 {"Timestamps"=[], "Phasor Data"=[], "Analog Data"=[], "Phasor Data 2"=[]}  # Data Cluster
              w159 = 0 ("index")
              n61 = First Call?() -> (First Call?: T/F=w155:bool)
              n62 = Unbundle By Name(w154) -> ("Timestamps"=w152:timestamp[], "Phasor Data"=w151:cdb[], "Analog Data"=w150:dbl[], "Phasor Data 2"=w149:cdb[])
              n63 = Unbundle By Name(w153) -> ("Timestamps"=w148:timestamp[], "Phasor Data"=w147:cdb[], "Analog Data"=w146:dbl[], "Phasor Data 2"=w145:cdb[])
              n64 = case shown="True" w155 {
                tunnel: [w167 w185] -> w135
                tunnel: [w166 w180] -> w156
                tunnel: [w165 w174] -> w157
                tunnel: w152 -> [w167 _]
                tunnel: w151 -> [w166 _]
                tunnel: w150 -> [w165 _]
                tunnel: [w164 w182] -> w127
                tunnel: [w163 w177] -> w129
                tunnel: [w162 w171] -> w124
                tunnel: w148 -> [w164 _]
                tunnel: w147 -> [w163 _]
                tunnel: w146 -> [w162 _]
                tunnel: [w161 w188] -> w134
                tunnel: [w160 w192] -> w158
                tunnel: w149 -> [w161 _]
                tunnel: w145 -> [w160 _]
                frame False {
                  # "Get the next set of values from the unused data set"
                }
                frame True {
                  w176 = 0 ("index")
                  n65 = local read "Signal Selection"() -> (w169:T7)
                  n66 = call "CSV_Reader_v1.vi"("CSV Reader Inputs"="CSV Reader Inputs") -> ("Terminals"=w196:T15[])  [unwired: 9 in, 1 out]
                  n67 = Equal?(x=w169, y=T7."Phase Comparison" ("Signal Selection")) -> (x = y?=w170:bool)
                  n68 = case shown="True" w170 {
                    tunnel: w196 -> [_ w200]
                    tunnel: [cdb[] [] ("Phasor Data") w198] -> w193
                    frame False {
                    }
                    frame True {
                      n69 = for {
                        tunnel: "Terminal ID 2 (Phase Comparison)" -> [w203]
                        tunnel: w200 -> [w205] mode=indexing
                        tunnel: [w202] -> w198
                        stop <- w201 stop-if-true
                        n70 = Unbundle By Name(w205) -> ("Terminal ID"=w204:dbl, "Phasor Data"=w202:cdb[])
                        n71 = Equal?(x=w204, y=w203) -> (x = y?=w201:bool)
                      }
                    }
                  }
                  n72 = for {
                    tunnel: "Terminal ID" -> [w215]
                    tunnel: w196 -> [w217] mode=indexing
                    tunnel: [w214] -> w187
                    tunnel: [w213] -> w181
                    tunnel: [w212] -> w175
                    tunnel: "CSV Reader Inputs" -> [w211]
                    stop <- w206 stop-if-true
                    n73 = Unbundle By Name(w217) -> ("Terminal ID"=w216:dbl, "Timestamps"=w214:timestamp[], "Phasor Data"=w213:cdb[], "Analog Data"=w212:dbl[])
                    n74 = Unbundle By Name(w211) -> ("Format Type"=w210:enum16{"Format A", "Format B"})
                    n75 = Equal?(x=w210, y=enum16{"Format A", "Format B"}."Format A" ("Format Type")) -> (x = y?=w208:bool)
                    n76 = Equal?(x=w216, y=w215) -> (x = y?=w207:bool)
                    n77 = Or(x=w208, y=w207) -> (x .or. y?=w206:bool)
                  }
                  n78 = Delete From Array(array=w187, index=0) -> (deleted portion=w184:timestamp, array with subset deleted=w185:timestamp[])  [unwired: 1 in]
                  n79 = Delete From Array(array=w181, index=w176) -> (deleted portion=w179:cdb, array with subset deleted=w180:cdb[])  [unwired: 1 in]
                  n80 = Delete From Array(array=w175, index=w176) -> (deleted portion=w173:dbl, array with subset deleted=w174:dbl[])  [unwired: 1 in]
                  n81 = Delete From Array(array=w193, index=0) -> (deleted portion=w191:cdb, array with subset deleted=w192:cdb[])  [unwired: 1 in]
                  n82 = Insert Into Array(array=timestamp[] [] ("Timestamps"), new element=w184) -> (w182:timestamp[])  [unwired: 1 in]
                  n83 = Insert Into Array(array=cdb[] [] ("Phasor Data"), new element=w179) -> (w177:cdb[])  [unwired: 1 in]
                  n84 = Insert Into Array(array=cdb[] [] ("Phasor Data"), new element=w191) -> (w188:cdb[])  [unwired: 1 in]
                  n85 = Insert Into Array(array=dbl[] [] ("Analog Data"), new element=w173) -> (w171:dbl[])  [unwired: 1 in]
                }
              }
              n86 = Delete From Array(array=w135, index=w159) -> (deleted portion=w126:timestamp, array with subset deleted=w143:timestamp[])  [unwired: 1 in]
              n87 = Delete From Array(array=w156, index=w159) -> (deleted portion=w130:cdb, array with subset deleted=w142:cdb[])  [unwired: 1 in]
              n88 = Delete From Array(array=w157, index=w159) -> (deleted portion=w123:dbl, array with subset deleted=w141:dbl[])  [unwired: 1 in]
              n89 = Delete From Array(array=w158, index=w159) -> (deleted portion=w133:cdb, array with subset deleted=w140:cdb[])  [unwired: 1 in]
              n90 = Bundle By Name(cluster=w144, "Timestamps"=w143, "Phasor Data"=w142, "Analog Data"=w141, "Phasor Data 2"=w140) -> (w139:T14)
              n91 = Insert Into Array(array=w127, new element=w126) -> (w128:timestamp[])  [unwired: 1 in]
              n92 = Insert Into Array(array=w129, new element=w130) -> (w131:cdb[])  [unwired: 1 in]
              n93 = Insert Into Array(array=w124, new element=w123) -> (w125:dbl[])  [unwired: 1 in]
              n94 = Array Size(array=w135) -> (size(s)=w137:i32)
              n95 = Insert Into Array(array=w134, new element=w133) -> (w132:cdb[])  [unwired: 1 in]
              n96 = Equal To 0?(x=w137) -> (x = 0?=w136:bool)
              n97 = Bundle By Name(cluster=w144, "Timestamps"=w128, "Phasor Data"=w131, "Analog Data"=w125, "Phasor Data 2"=w132) -> (w138:T14)
            }
          }
          n98 = case shown="\"Analog\"" "Signal Selection" {
            tunnel: [w218 w228 w230 w232 w234] -> w90
            tunnel: w91 -> [w226 _ w231 w233 w235]
            tunnel: w93 -> [_ w227 _ _ _]
            tunnel: w89 -> [w221 _ _ _ _]
            frame "Phase Comparison" {
              w222 = 0 items=["radian in, radian out", "radian in, degree out", "degree in, degree out", "degree in, radian out"] ("phase unit")
              w225 = 0 items=["radian in, radian out", "radian in, degree out", "degree in, degree out", "degree in, radian out"] ("phase unit")
              n99 = Complex To Polar(r * e^(i*theta)=w221) -> (theta=w223:dbl[])  [unwired: 1 out]
              n100 = Complex To Polar(r * e^(i*theta)=w226) -> (theta=w224:dbl[])  [unwired: 1 out]
              n101 = call <vilib>:"Unwrap Phase.vi"("phase unit"=w222, "Phase"=w223) -> ("Unwrapped Phase"=w219:dbl[])  [unwired: 8 in, 1 out]
              n102 = call <vilib>:"Unwrap Phase.vi"("phase unit"=w225, "Phase"=w224) -> ("Unwrapped Phase"=w220:dbl[])  [unwired: 8 in, 1 out]
              n103 = Subtract(x=w220, y=w219) -> (x-y=w218:dbl[])
            }
            frame "Analog" {
              n104 = To Double Precision Float(number=w227) -> (double precision float=w228:dbl[])
            }
            frame "Mag", Default {
              n105 = Complex To Polar(r * e^(i*theta)=w231) -> (r=w229:dbl[])  [unwired: 1 out]
              n106 = To Double Precision Float(number=w229) -> (double precision float=w230:dbl[])
            }
            frame "Imaginary Component" {
              n107 = Complex To Re/Im(x + iy=w233) -> (y=w232:dbl[])  [unwired: 1 out]
            }
            frame "Real Component" {
              n108 = Complex To Re/Im(x + iy=w235) -> (x=w234:dbl[])  [unwired: 1 out]
            }
          }
          n109 = local read "Sampling Frequency (Hz)"() -> (w101:dbl)
          n110 = local read "Test Method"() -> (w76:enum16{"Use PRL Data", "Read from CSV File"})
          n111 = Reciprocal(x=w101) -> (1/x=w78:dbl)
          n112 = local read "MA Order"() -> (w100:i32)
          n113 = local read "AR Order"() -> (w102:i32)
          n114 = Index Array "Index Array"(array=w94, index #1=0 ("index"), index #2=1 ("index")) -> (element #1=w79:timestamp, element #2=w80:timestamp)
          n115 = case shown="\"Read from CSV File\"" w76 {
            tunnel: w80 -> [_ w109]
            tunnel: w79 -> [_ w108]
            tunnel: w78 -> [w104 _]
            tunnel: [w104 w107] -> w77
            frame "Use PRL Data" {
              # "Use sampling frequency\nfor period"
            }
            frame "Read from CSV File" {
              n116 = To Extended Precision Float(1:w108) -> (0:w105:ext)
              n117 = To Extended Precision Float(1:w109) -> (0:w106:ext)
              n118 = Subtract(x=w106, y=w105) -> (x-y=w107:ext)
            }
          }
          n119 = Array Size(array=w90) -> (size(s)=w95:i32)
          n120 = Bundle By Name("t0"=w79, "dt"=w77, "Y"=w90) -> (w103:waveform(dbl))  [unwired: 1 in]
          n121 = Bundle By Name(cluster=w86, "Waveform"=w103, "Parcel Length"=w95, "Sampling Frequency"=w101, "AR Order"=w102, "MA Order"=w100) -> (w96:T9)
        }
        frame "Read Simulated Data" {
          w243 = "H"
          # "Enter data into the Data cluster"
          n122 = case shown="\"Use Input Poles/Zeroes\"" "Simulation Method" {
            tunnel: [dbl[] [1.0] ("Array") w295] -> w241
            tunnel: [w289 w297] -> w240
            frame "Use Input Frequency/D.R." {
              w274 = T8."Disabled and Grayed Out" ("Disabled")
              n123 = Multiply(x=2.0 ("y"), y=3.141592653589793) -> (x*y=w291:dbl)
              n124 = Multiply(x="Input Frequency (Hz)", y=w291) -> (x*y=w287:dbl)
              n125 = Divide(x="Input Damping Ratio (%)", y=100.0) -> (x/y=w277:dbl)
              n126 = Square(x=w287) -> (x^2=w286:dbl)
              n127 = Square(x=w277) -> (x^2=w280:dbl)
              n128 = Subtract(x=1.0 ("standard deviation"), y=w280) -> (x-y=w279:dbl)
              n129 = Divide(x=w286, y=w279) -> (x/y=w278:dbl)
              n130 = Square Root(x=w278) -> (sqrt(x)=w282:dbl)
              n131 = Multiply(x=w282, y=w277) -> (x*y=w283:dbl)
              n132 = Multiply(x=w283, y=2.0) -> (x*y=w285:dbl)
              n133 = property on="Input Zeros" class="Arr (strict)"("DisabledEnum"=w274) -> ()  [unwired: 2 in, 2 out]
              n134 = Build Array(w278, w285, 1.0 ("standard deviation")) -> (w289:dbl[])
              n135 = property on="Input Poles" class="Arr (strict)"("DisabledEnum"=w274) -> ()  [unwired: 2 in, 2 out]
            }
            frame "Use Input Poles/Zeroes" {
              w299 = T8."Disabled and Grayed Out" ("Disabled")
              n136 = mathscript code="[num, den] = zpk_to_tf(zeros, poles, 1)"("zeros"="Input Zeros", "poles"="Input Poles") -> ("num"=w296:dbl[], "den"=w298:dbl[])  [unwired: 1 in, 1 out]
              n137 = property on="Input Frequency (Hz)" class="DigNum (strict)"("DisabledEnum"=w299) -> ()  [unwired: 2 in, 2 out]
              n138 = property on="Input Damping Ratio (%)" class="DigNum (strict)"("DisabledEnum"=w299) -> ()  [unwired: 2 in, 2 out]
              n139 = Reverse 1D Array(array=w298) -> (reversed array=w297:dbl[])
              n140 = Reverse 1D Array(array=w296) -> (reversed array=w295:dbl[])
            }
          }
          n141 = call <vilib>:"Gaussian White Noise.vi"("standard deviation"=10.0, "samples"="Parcel Length (Simulation)") -> ("Gaussian noise pattern"=w262:dbl[])  [unwired: 8 in, 1 out]
          n142 = Reshape Array "Reshape Array"(w262, 1 ("dimension size"), 30000 ("dimension size")) -> (w261:dbl[][])
          n143 = call-poly <vilib>:"CD Construct Transfer Function Model.vi"("Denominator"=w240, "Numerator"=w241) -> ("error out"=w244:errorcluster, "Transfer Function Model"=w246:T16)  [unwired: 8 in]
          n144 = call-poly <vilib>:"CD Set Names to Model.vi"("Model Name"=w243, "Transfer Function Model In"=w246, "error in (no error)"=w244) -> ("Model Out"=w239:T16, "error out"=w245:errorcluster)  [unwired: 11 in]
          n145 = call-poly <vilib>:"CD Draw Transfer Function Equation.vi"("Function Name (empty)"=w243, "error in (no error)"=w245, "Transfer Function Model"=w239) -> ("error out"=w242:errorcluster, "Equation"=→"Input Transfer Function":picture)  [unwired: 6 in, 1 out]
          n146 = call-poly <vilib>:"CD Linear Simulation.vi"("Delta t"=0.02, "error in (no error)"=w242, "Inputs"=w261, "Transfer Function Model"=w239) -> ("Simulation Data"=w260:T19)  [unwired: 5 in, 2 out]
          n147 = Unbundle By Name(w260) -> ("Outputs Data"=w257:dbl[][][])
          n148 = call-poly <vilib>:"CD Damping Ratio and Natural Frequency.vi"("Transfer Function Model"=w239) -> ("Poles"=→"Poles":cdb[], "Natural Frequencies"=→"Natural Frequencies":dbl[], "Damping Ratios"=w251:dbl[])  [unwired: 7 in, 1 out]
          n149 = To Double Precision Float(number=100 ("length")) -> (double precision float=w248:dbl)
          n150 = Multiply(x=w248, y=w251) -> (x*y=→"Damping Ratios (%)":dbl[])
          n151 = Get Date/Time In Seconds() -> (seconds since 1Jan1904=w264:timestamp)
          n152 = Index Array "Index Array"(array=w257, index (dim 0)=0 ("index"), index (dim 2)=0 ("length")) -> (element=w255:dbl[])  [unwired: 1 in]
          n153 = Reciprocal(x="Sampling Frequency (Hz)") -> (1/x=w269:dbl)
          n154 = Bundle By Name("t0"=w264, "dt"=w269, "Y"=w255) -> (w270:waveform(dbl))  [unwired: 1 in]
          n155 = Bundle By Name(cluster=w273, "Waveform"=w270, "Parcel Length"="Parcel Length (Simulation)", "Sampling Frequency"="Sampling Frequency (Hz)", "AR Order"="AR Order", "MA Order"="MA Order") -> (w265:T9)
        }
        frame "Preprocessing" {
          # "New Waveform and Frequency"
          # "Detrend the transfer function, pass it through a LPF, then rescale it (downsample)"
          n156 = Unbundle By Name(w371) -> ("Waveform"=w373:waveform(dbl), "Sampling Frequency"=w375:dbl, "Parcel Length"=→"Parcel Length (SDK or Simulation)":i32)
          n157 = call-poly <vilib>:"WA Detrend.vi"("threshold frequency"="Detrend Cut-off Frequency (Hz)", "signal"=w373) -> ("detrended signal"=w376:waveform(dbl))  [unwired: 7 in, 2 out]
          n158 = call-poly "SI Lowpass Filter.vi"("cutoff frequency"="LPF Cut-off Frequency [Hz]", "order"="Low-Pass Filter Order", "stimulus signal in"=w376) -> ("stimulus signal out"=w365:waveform(dbl))  [unwired: 6 in, 2 out]
          n159 = To Long Integer(number="Downsampling Ratio") -> (32bit integer=w364:i32)
          n160 = call "Downsample v1.vi"("Divide by"=w364, "Waveform in"=w365) -> ("Waveform out"=w363:waveform(dbl))  [unwired: 9 in]
          "Preprocessed data" <- w363
          n161 = Divide(x=w375, y="Downsampling Ratio") -> (x/y=w374:dbl)
          n162 = Bundle By Name(cluster=w371, "Waveform"=w363, "Sampling Frequency"=w374) -> (w380:T9)
        }
        frame "Compute AR/MA Coeffs" {
          w440 = T21 5 items=["Zero-Order-Hold", "Tustin (Bilinear)", "Prewarp", "Forward", "Backward", "Z-Transform"] ("Method")
          w443 = u16 0 items=["Yule-Walker", "High order AR", "Polynomial"] ("method")
          # "Convert back into s-domain"
          # "Eliminates the poles that have negative/0 complex component,\nand eliminates duplicate frequencies/damping ratios and those \noutside of the bounds (as per the lower/upper values)"
          n163 = control-ref of="Estimated Complex Plane"() -> (w434:refnum<vi>)
          n164 = Unbundle By Name(w442) -> ("Waveform"=w441:waveform(dbl), "AR Order"=w439:i32, "MA Order"=w405:i32, "Sampling Frequency"=w403:dbl)
          n165 = property class="XYGraph (strict)"(reference=w434, "BG Color"=u32 16448250 ("Color Box")) -> ()  [unwired: 1 in, 2 out]
          n166 = Bundle("AR Order"=w439, "MA Order"=w405) -> (w438:cluster{"AR Order":i32, "MA Order ":i32})  [unwired: 1 in]
          n167 = Reciprocal(x=w403) -> (1/x=w404:dbl)
          n168 = call-poly <vilib>:"TSA ARMA Modeling.vi"("ARMA order"=w438, "method"=w443, "Xt"=w441) -> ("error out"=w387:errorcluster, "MA coefficients"=w393:dbl[], "AR coefficients"=w396:dbl[])  [unwired: 5 in, 1 out]
          n169 = Reverse 1D Array(array=w396) -> (reversed array=w420:dbl[])
          n170 = Reverse 1D Array(array=w393) -> (reversed array=w421:dbl[])
          n171 = call-poly <vilib>:"CD Construct Transfer Function Model.vi"("Sampling Time (s)"=w404, "error in (no error)"=w387, "Denominator"=w420, "Numerator"=w421) -> ("error out"=w389:errorcluster, "Transfer Function Model"=w392:T16)  [unwired: 6 in]
          n172 = call-poly <vilib>:"CD Draw Transfer Function Equation.vi"("Function Name (empty)"="   B(z) / A", "error in (no error)"=w389, "Transfer Function Model"=w392) -> ("error out"=w388:errorcluster, "Equation"=→"ARMA Transfer Function":picture)  [unwired: 6 in, 1 out]
          n173 = call-poly <vilib>:"CD Convert Discrete to Continuous.vi"("error in (no error)"=w388, "Method"=w440, "Discrete Transfer Function Model"=w392) -> ("error out"=w415:errorcluster, "Continuous Transfer Function Model"=w409:T16)  [unwired: 7 in]
          n174 = call-poly <vilib>:"CD Convert to State-Space Model.vi"("error in (no error)"=w415, "Realization Type"=enum16{"minimum", "full"}."full", "Transfer Function Model"=w409) -> ("error out"=w408:errorcluster, "State-Space Model"=w413:T22)  [unwired: 7 in]
          n175 = call-poly <vilib>:"CD Damping Ratio and Natural Frequency.vi"("error in (no error)"=w408, "Frequency Unit"=enum16{"Hz", "rad/s"}."Hz", "State-Space Model"=w413) -> ("Poles"=w422:cdb[], "Natural Frequencies"=w416:dbl[], "Damping Ratios"=w428:dbl[])  [unwired: 5 in, 1 out]
          n176 = To Double Precision Float(number=100 ("Numeric")) -> (double precision float=w407:dbl)
          n177 = Multiply(x=w407, y=w428) -> (x*y=w426:dbl[])
          n178 = mathscript code="[damp,ind]=sort(damp);\nfreq=freq(ind);\npoles=poles(ind);\n\nind=find(freq>LowF & freq<UpF & damp>LowD & damp<UpD &  imag(poles)>=0)\ndamp=damp(ind)\nfreq=freq(ind);\npoles=poles(ind);"("damp"=w426, "freq"=w416, "poles"=w422, "LowF"="Lower Frequency [Hz]", "UpF"="Upper Frequency [Hz]", "LowD"="Lower Damping [%]", "UpD"="Upper Damping [%]") -> ("poles"=w412:cdb[], "freq"=w395:dbl[], "damp"=w394:dbl[])  [unwired: 1 in, 1 out]
          "Complex Poles" <- w412
          "Frequency[Hz]" <- w395
          "Damping Ratio [%]" <- w394
          n179 = Build Array (concatenate) "Build Array"(w394, w432) -> (w402:dbl[][])
          n180 = local read "Length of Spectra [s]"() -> (w427:dbl)
          n181 = Complex To Re/Im(x + iy=w412) -> (x=w437:dbl[], y=w436:dbl[])
          n182 = Bundle(w437, w436) -> (→"Estimated Complex Plane":cluster{dbl[], dbl[]})  [unwired: 1 in]
          n183 = Array Subset "Array Subset"(array=w402, index (row)=0 ("index"), length (row)=w427, index (col)=0 ("index"), length (col)="Number of critical modes") -> (w401:dbl[][])
          n184 = Transpose 2D Array(2D array=w401) -> (transposed array=→"Damping ratio evolution":dbl[][])
          n185 = for {
            N: "Number of critical modes" -> [_]
            tunnel: w402 -> [w459]
            tunnel: [w457] -> w425 mode=indexing
            tunnel: [w456] -> w384 mode=indexing
            i -> [w455]
            # "Take Std. Deviation and Mean\nof Damping Ratios"
            n186 = Index Array "Index Array"(array=w459, index (col)=w455) -> (element=w458:dbl[])  [unwired: 1 in]
            n187 = call <vilib>:"Std Deviation and Variance.vi"("X"=w458, "Weighting (Sample)"=enum16{"Sample", "Population"}."Sample") -> ("mean"=w457:dbl, "standard deviation"=w456:dbl)  [unwired: 1 out]
          }
          "Std of Damping" <- w384
          "Mean Damping [%]" <- w425
          n188 = Index Array(array=w395, index=0) -> (element=→"Critical Frequency [Hz]":dbl)
          n189 = call "smiley v1.vi"("std threshold"="Std Threshold", "damp"=w384) -> ("Array"=w382:picture[])  [unwired: 9 in]
          n190 = for {
            tunnel: w382 -> [w444] mode=indexing
            i -> [w445]
            n191 = case shown="0, Default" w445 {
              tunnel: w444 -> [w446 w447 w448 w449 w450 w451 w452 w453 w454]
              frame 0, Default {
                "Picture 1" <- w446
              }
              frame 1 {
                "Picture 2" <- w447
              }
              frame 2 {
                "Picture 3" <- w448
              }
              frame 3 {
                "Picture 4" <- w449
              }
              frame 4 {
                "Picture 5" <- w450
              }
              frame 5 {
                "Picture 6" <- w451
              }
              frame 6 {
                "Picture 7" <- w452
              }
              frame 7 {
                "Picture 8" <- w453
              }
              frame 8 {
                "Picture 9" <- w454
              }
            }
          }
          n192 = Index Array(array=w394, index=0 ("length")) -> (element=→"Critical Damping [%]":dbl)
        }
        frame "Get Spectrum" {
          w702 = u16 0 items=["Yule-Walker", "High order AR", "Polynomial"] ("method")
          # "Continue to read the data"
          n193 = local read "Refresh Rate [s]"() -> (w687:i32)
          n194 = Unbundle By Name(w700) -> ("Waveform"=w712:waveform(dbl), "AR Order"=w715:i32, "MA Order"=w714:i32)
          n195 = Bundle("AR Order"=w715, "MA Order"=w714) -> (w713:cluster{"AR Order":i32, "MA Order ":i32})  [unwired: 1 in]
          n196 = call-poly <vilib>:"TSA ARMA Spectrum.vi"("dB on? (T)"="dB Scale", "ARMA order"=w713, "method"=w702, "Xt"=w712) -> ("PSD"=w701:cluster{"f0":dbl, "df":dbl, "S(f)":dbl[]})  [unwired: 5 in, 2 out]
          "Spectrum" <- w701
          n197 = To Double Precision Float(number=w687) -> (double precision float=w688:dbl)
          n198 = Unbundle By Name(w701) -> ("f0"=w710:dbl, "df"=w709:dbl, "S(f)"=w706:dbl[])
          n199 = Quotient & Remainder(x="Length of Spectra [s]", y=w688) -> (floor(x/y)=w690:dbl)  [unwired: 1 out]
          n200 = Increment(x=w690) -> (x+1=w689:dbl)
          n201 = for {
            tunnel: w706 -> [_] mode=indexing
            tunnel: w710 -> [w719]
            tunnel: w709 -> [w721]
            tunnel: [w718] -> w698 mode=indexing
            i -> [w722]
            n202 = Decrement(x=w722) -> (x-1=w716:i32)
            n203 = To Double Precision Float(number=w716) -> (double precision float=w717:dbl)
            n204 = Multiply(x=w721, y=w717) -> (x*y=w720:dbl)
            n205 = Add(x=w719, y=w720) -> (x+y=w718:dbl)
          }
          n206 = feedback #1(dbl[] [] ("XX")) -> (w708:dbl[])
          n207 = feedback #2(0.0 ("i")) -> (w711:dbl)
          n208 = feedback #3(0.0 ("TDold")) -> (w694:dbl)
          n209 = feedback #4(dbl[][] [] ("Array")) -> (w704:dbl[][])
          n210 = mathscript code="if (TDold ~=TimeDiff)\ni=0\nend\nif i>Limit\nXX=XX(i-Limit+1:i);\ni=Limit;\nend\nif i==Limit\nArray=Array(2:i,:);\nArray(i,:)=Data(:);\nelse\ni=i+1\nArray(i,:)=Data(:);\nXX(i)=0;\n\nif i==1\nXX(1)=0;\nelse\nXX(1:i-1)=XX(1:i-1)-TimeDiff\nXX(i)=0\nend\nend\n\nTDold=TimeDiff;"("Data"=w706, "Array"=w704, "i"=w711, "Limit"=w689, "XX"=w708, "TimeDiff"=w687, "TDold"=w694) -> ("Array"=w697:dbl[][], "i"=w685:dbl, "XX"=w695:dbl[], "TDold"=w682:i32)  [unwired: 1 in, 1 out]
          n211 = feedback-in #1(w695) -> ()
          n212 = feedback-in #2(w685) -> ()
          n213 = To Double Precision Float(number=w682) -> (double precision float=w683:dbl)
          n214 = feedback-in #3(w683) -> ()
          n215 = feedback-in #4(w697) -> ()
          n216 = call-poly <vilib>:"Plot Helper.vi"("z matrix"=w697, "y vector"=w698, "x vector"=w695) -> ("3D Plot lvclass Array out"=→"Spectrogram":refnum<class "3D Plot Datatype.lvclass">[])  [unwired: 3 in, 5 out]
          n217 = local read "Simulation"() -> (w699:bool)
          n218 = Select(t=State."Read Simulated Data" ("Enum"), s=w699, f=State."Read Real Data" ("Enum")) -> (s? t:f=w681:T10)
        }
      }
      n219 = local read "Refresh Rate [s]"() -> (w52:i32)
      n220 = Multiply(x=w52, y=1000) -> (x*y=w41:i32)
      n221 = To Double Precision Float(number=w41) -> (double precision float=w42:dbl)
      n222 = Divide(x=w42, y=4.0) -> (x/y=w53:dbl)
      n223 = To Quad Integer(1:w53) -> (0:w50:i64)
      n224 = Not Equal?(x=w50, y=w56) -> (x != y?=w33:bool)
      n225 = Or(x=w32, y=w33) -> (x .or. y?=w31:bool)
      n226 = Or(x=w31, y="stop") -> (x .or. y?=w34:bool)
      n227 = Unbundle By Name(w44) -> ("Waveform"=→"Real-time data":waveform(dbl))
      n228 = node-c288() -> ()  [unwired: 1 in, 1 out]
    }
    n229 = node-c288(w19) -> ()  [unwired: 1 out]
  }
